vi "ReduceArray.vi"(11 "I/P Array":dbl[](array[numeric])) -> (3 "Reduced Array":dbl[](array[numeric]))   [LabVIEW 2017]
uses:
  GlobalVariables.vi
panel:
  # "This function reduces an input array from dimension 8 to \nno. of motors in use as per motor selection.\nIt can be used with all sensors values."
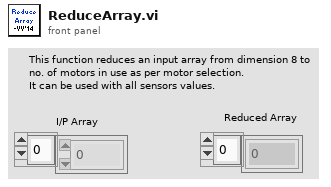
[diagram p1: front panel]
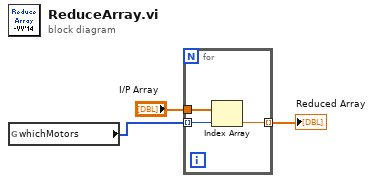
[diagram p0: block diagram]
diagram:
  n1 = global read "GlobalVariables.vi" "whichMotors"() -> (w1:i32[])
  n2 = for {
    tunnel: w1 -> [w6] mode=indexing
    tunnel: [w5] -> w3 mode=indexing
    tunnel: "I/P Array" -> [w4]
    n3 = Index Array(array=w4, index=w6) -> (element=w5:dbl)
  }
  "Reduced Array" <- w3
